vi "KB-Cal-Distance.vi"(10 "Fitted Circle (Inner Find Circular Edge 2)":T1, 11 "Fitted Circle (Otter-Find Circular Edge)":T1) -> (3 "Distance":sgl)   [LabVIEW 2015]
panel:
  in  "Row Select":string(combo)="Item1"
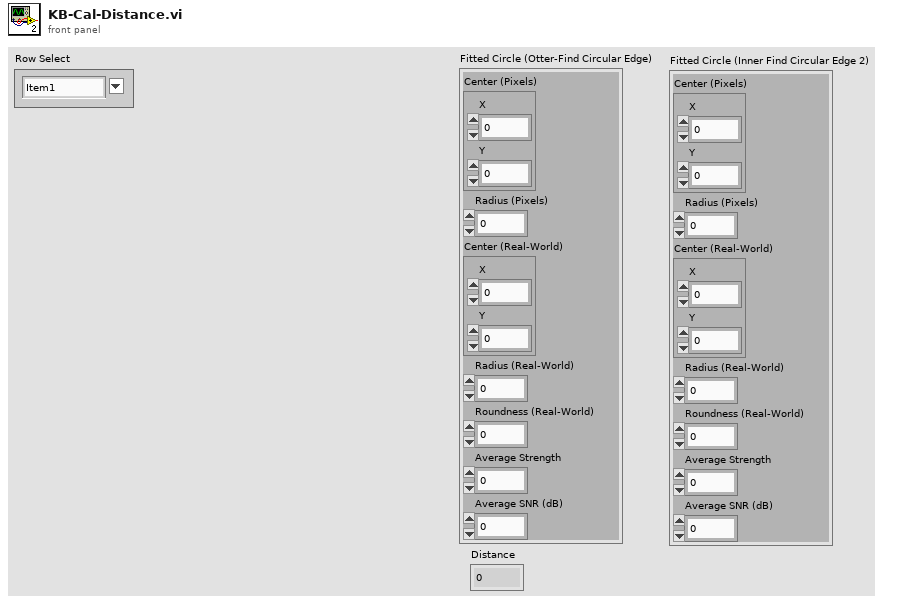
[diagram p1: front panel]
types:
  T1 = cluster{"Center (Pixels)":cluster{"X":sgl, "Y":sgl}, "Radius (Pixels)":dbl, "Center (Real-World)":cluster{"X":sgl, "Y":sgl}, "Radius (Real-World)":dbl, "Roundness (Real-World)":dbl, "Average Strength":dbl, "Average SNR (dB)":dbl}
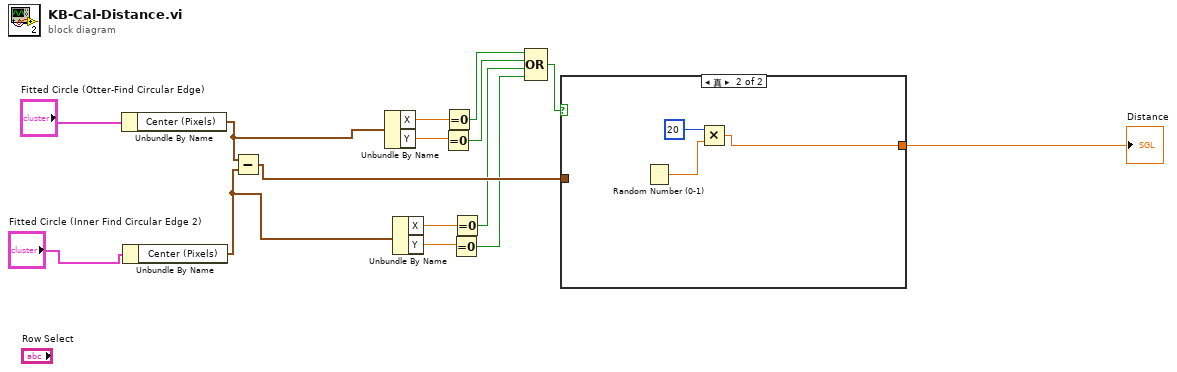
[diagram p0: block diagram]
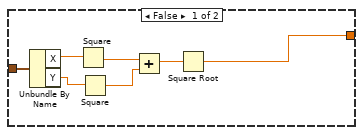
[diagram p2: hidden frame]
diagram:
  n1 = Unbundle By Name("Fitted Circle (Otter-Find Circular Edge)") -> ("Center (Pixels)"=w11:cluster{"X":sgl, "Y":sgl})
  n2 = Unbundle By Name("Fitted Circle (Inner Find Circular Edge 2)") -> ("Center (Pixels)"=w6:cluster{"X":sgl, "Y":sgl})
  n3 = Subtract(x=w11, y=w6) -> (x-y=w13:cluster{"X":sgl, "Y":sgl})
  n4 = Unbundle By Name(w11) -> ("X"=w10:sgl, "Y"=w9:sgl)
  n5 = Unbundle By Name(w6) -> ("X"=w7:sgl, "Y"=w8:sgl)
  n6 = Equal To 0?(x=w9) -> (x = 0?=w4:bool)
  n7 = Equal To 0?(x=w10) -> (x = 0?=w5:bool)
  n8 = Equal To 0?(x=w8) -> (x = 0?=w2:bool)
  n9 = Equal To 0?(x=w7) -> (x = 0?=w3:bool)
  n10 = Compound Arithmetic op=OR ("复合运算")(w5, w4, w3, w2) -> (w1:bool)
  n11 = case shown="真" w1 {
    tunnel: w13 -> [w22 _]
    tunnel: [w16 w23] -> w12
    frame False {
      n12 = Unbundle By Name(w22) -> ("X"=w21:sgl, "Y"=w20:sgl)
      n13 = Square(x=w21) -> (x^2=w19:sgl)
      n14 = Square(x=w20) -> (x^2=w18:sgl)
      n15 = Add(x=w19, y=w18) -> (x+y=w17:sgl)
      n16 = Square Root(x=w17) -> (sqrt(x)=w16:sgl)
    }
    frame True {
      n17 = Random Number (0-1)() -> (number: 0 to 1=w24:dbl)
      n18 = Multiply(x=20, y=w24) -> (x*y=w23:dbl)
    }
  }
  "Distance" <- w12
